vi "gas gesteuert.vi"   [LabVIEW 2016]
uses:
  <vilib>/dex/Stream Element Allocation Mode.ctl
  <vilib>/myRIO/Instrument Drivers/Onboard IO/PWM/typedefs/PWM Reference.ctl
  <vilib>/myRIO/Common/Instrument Driver Framework/Utilities/typedefs/myRIO Generic Hardware Reference.ctl
  <vilib>/myRIO/Common/Instrument Driver Framework/Utilities/typedefs/Hardware Version Enum.ctl
  <vilib>/myRIO/Common/Instrument Driver Framework/Utilities/typedefs/myRIO v1.0 Reference.ctl
  <vilib>/myRIO/Common/Instrument Driver Framework/Utilities/typedefs/Generic FPGA Reference.ctl
  <vilib>/myRIO/Common/Instrument Driver Framework/myRIO v1.0/PWM/typedefs/PWM Channels Enum.ctl
  <vilib>/myRIO/Instrument Drivers/Onboard IO/PWM/typedefs/PWM Configuration.ctl
  <vilib>/userdefined/High Color/nirio_resource_hc.ctl
  <vilib>/myRIO/Common/Instrument Driver Framework/Utilities/vis/Is FPGA Ref Available.vi
  <vilib>/myRIO/Common/Instrument Driver Framework/myRIO v1.0/PWM/vis/myRIO v1.1 Open PWM.vi
  <vilib>/myRIO/Instrument Drivers/Onboard IO/PWM/vis/Set Duty Cycle and Frequency.vi
  <vilib>/myRIO/Common/Instrument Driver Framework/Utilities/vis/Validate Channels.vi
  <vilib>/myRIO/Common/Instrument Driver Framework/myRIO v1.0/PWM/vis/myRIO v1.0 Reserve PWM.vi
  <vilib>/myRIO/Common/Instrument Driver Framework/myRIO v1.0/PWM/vis/myRIO v1.0 Build MUX Configuration PWM.vi
  <vilib>/myRIO/Common/Instrument Driver Framework/myRIO v1.0/Resource Manager/vis/myRIO v1.0 Reserve Channel List.vi
  <vilib>/myRIO/Common/Instrument Driver Framework/myRIO v1.0/Resource Manager/vis/myRIO v1.0 Create Configuration List.vi
  <vilib>/myRIO/Common/Instrument Driver Framework/myRIO v1.0/Resource Manager/vis/myRIO v1.0 Reserve Channel.vi
  <vilib>/myRIO/Common/Instrument Driver Framework/myRIO v1.0/Resource Manager/vis/myRIO v1.0 Unreserve Channel.vi
  <vilib>/myRIO/Common/Instrument Driver Framework/myRIO v1.0/Resource Manager/vis/myRIO v1.0 Build Mutex Name.vi
  <vilib>/Utility/VariantDataType/GetNumericInfo.vi
  <vilib>/Utility/error.llb/Error Cluster From Error Code.vi
  <vilib>/myRIO/Common/Instrument Driver Framework/myRIO v1.0/myRIO v1.1 Open.vi
  <vilib>/myRIO/Common/Instrument Driver Framework/Utilities/vis/IO Manager.vi
  <vilib>/myRIO/Common/Instrument Driver Framework/Utilities/vis/Configuration Manager.vi
  <vilib>/myRIO/Common/Instrument Driver Framework/myRIO v1.0/Resource Manager/vis/myRIO v1.0 Configure IO.vi
  <vilib>/myRIO/Common/Instrument Driver Framework/myRIO v1.0/myRIO v1.0 Close.vi
  <vilib>/myRIO/Common/Instrument Driver Framework/myRIO v1.0/PWM/vis/myRIO v1.0 Write PWM.vi
  <vilib>/myRIO/Express VI/Onboard IO/PWM/PWM Express VI.xnode
  <vilib>/myRIO/Instrument Drivers/Onboard IO/PWM/vis/myRIO PWM Open.xnode
  <vilib>/myRIO/Instrument Drivers/Onboard IO/PWM/PWM.lvlib
types:
  T1 = typedef "Stream Element Allocation Mode.ctl" = u32
  T2 = typedef "PWM.lvlib/PWM Reference.ctl" = cluster{"myRIO Reference":T3, "PWM Channels Enum":T7, "PWM Configuration":T8}
  T3 = typedef "myRIO Generic Hardware Reference.ctl" = cluster{"myRIO Model":T4, "myRIO Hardware Reference":T5}
  T4 = typedef "Hardware Version Enum.ctl" = enum16{"Unknown", "myRIO-1900", "myRIO-1950", "roboRIO", "NI ELVIS RIO CM"}
  T5 = typedef "myRIO v1.0 Reference.ctl" = cluster{"Generic FPGA Reference":T6, "Allow multiple opens":bool}
  T6 = typedef "Generic FPGA Reference.ctl" = refnum<k20>
  T7 = typedef "PWM Channels Enum.ctl" = enum16{"Not Connected", "C/PWM0", "C/PWM1", "A/PWM0", "A/PWM1", "A/PWM2", "B/PWM0", "B/PWM1", "B/PWM2", "PWM/PWM0", "PWM/PWM1", "PWM/PWM2", "PWM/PWM3", "PWM/PWM4", "PWM/PWM5", "PWM/PWM6", "PWM/PWM7", "PWM/PWM8", "PWM/PWM9"}
  T8 = typedef "PWM.lvlib/PWM Configuration.ctl" = cluster{"Frequency":dbl, "Duty Cycle":dbl}
  T9 = typedef "nirio_resource_hc.ctl" = tag
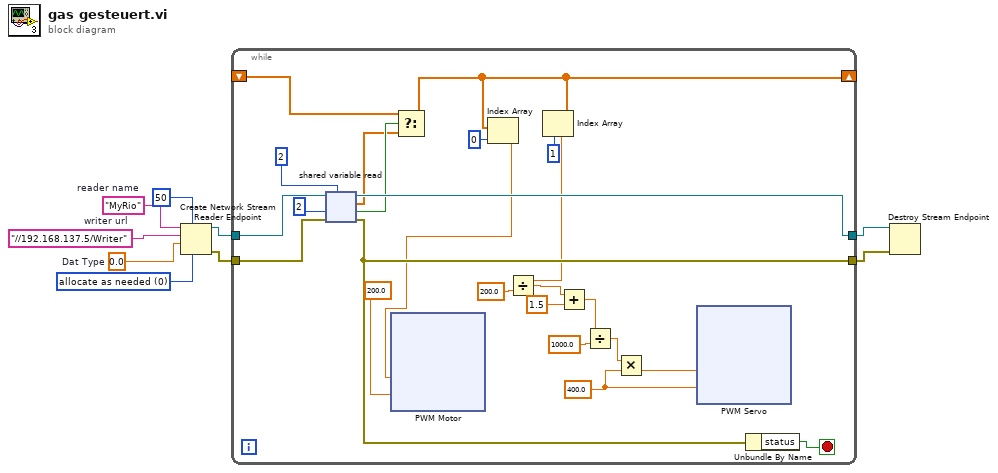
[diagram p0: block diagram]
diagram:
  w3 = T1 0 items=["allocate as needed", "pre-allocate"] ("element allocation mode")
  w4 = "//192.168.137.5/Writer"  # writer url
  w8 = 0.0  # Dat Type
  w9 = "MyRio"  # reader name
  n1 = Create Network Stream Reader Endpoint(6:w3, 7:50 ("reader buffer size"), 9:w8, 10:w4, 11:w9) -> (0:w2:errorcluster, 3:w1:refnum<k21>)  [unwired: 2 in]
  n2 = while {
    shift-right: [w12] -> _
    shift-left: _ -> [w14]
    tunnel: w1 -> [w16]
    tunnel: [w30] -> w6
    tunnel: w2 -> [w17]
    tunnel: [w31] -> w7
    stop <- w32 stop-if-true
    w21 = 400.0 ("Frequency [Hz]")
    n3 = shared-variable-read ("Read Multiple Elements from Stream")(w16, w17, 2 ("timeout ms (-1)"), 2 ("# elements")) -> (w30:refnum<k21>, w31:errorcluster, w15:bool, w13:dbl[])
    n4 = Select(t=w14, s=w15, f=w13) -> (s? t:f=w12:dbl[])
    n5 = Index Array(array=w12, index=0) -> (element=w28:dbl)
    n6 = xnode "PWM Motor"("Duty Cycle"=w28, "Frequency [Hz]"=200.0) -> ()  [unwired: 1 in, 1 out]
    n7 = Index Array(array=w12, index=1) -> (element=w19:dbl)
    n8 = Divide(x=w19, y=200.0) -> (x/y=w26:dbl)
    n9 = Add(x=w26, y=1.5) -> (x+y=w24:dbl)
    n10 = Divide(x=w24, y=1000.0) -> (x/y=w22:dbl)
    n11 = Multiply(x=w22, y=w21) -> (x*y=w20:dbl)
    n12 = xnode "PWM Servo"("Duty Cycle"=w20, "Frequency [Hz]"=w21) -> ()  [unwired: 1 in, 1 out]
    n13 = Unbundle By Name "Unbundle By Name"(w31) -> ("status"=w32:bool)
  }
  n14 = Destroy Stream Endpoint(8:w7, 11:w6) -> ()  [unwired: 1 out]
